vi "RSZVB Get Sweep Segment Name.vi"(8 "error in (no error)":errorcluster {"code" format="%.0x"}, 9 "Segment (1)":i32=1, 10 "Channel (1)":i32=1, 11 "VISA session":refnum<visa-resource-name>) -> (0 "error out":errorcluster {"code" format="%.0x"}, 2 "Name":string, 3 "dup VISA session":refnum<visa-resource-name>)   [LabVIEW 2011]
doc: "This VI returns the Name of the sweep segment no. <Seg>.\n\nRemote-control command(s):\n[SENSe<Ch>:]SEGMent<Seg>:NAME?"
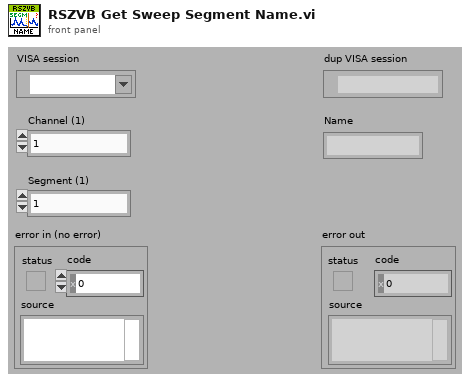
[diagram p1: front panel]
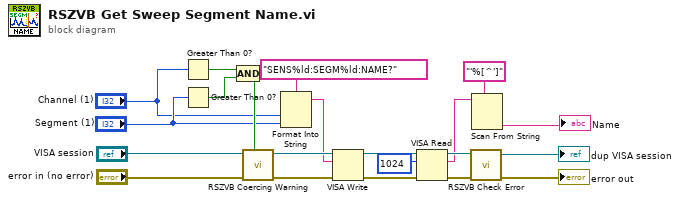
[diagram p0: block diagram]
diagram:
  n1 = Greater Than 0?(x="Channel (1)") -> (x > 0?=w16:bool)
  n2 = Greater Than 0?(x="Segment (1)") -> (x > 0?=w15:bool)
  n3 = Compound Arithmetic op=AND(w16, w15) -> (w18:bool)
  n4 = call "RSZVB Coercing Warning.vi"("In Range?"=w18, "error in (no error)"="error in (no error)", "VISA session"="VISA session") -> ("error out"=w19:errorcluster, "dup VISA session"=w20:refnum<visa-resource-name>)  [unwired: 7 in]
  n5 = Format Into String(format string="SENS%ld:SEGM%ld:NAME?", "Channel (1)", "Segment (1)") -> (resulting string=w17:string)  [unwired: 2 in, 1 out]
  n6 = VISA Write(VISA resource name=w20, write buffer=w17, error in (no error)=w19) -> (VISA resource name out=w11:refnum<visa-resource-name>, error out=w10:errorcluster)  [unwired: 1 out]
  n7 = VISA Read(VISA resource name=w11, byte count=u32 1024 ("byte count (0)"), error in (no error)=w10) -> (VISA resource name out=w13:refnum<visa-resource-name>, read buffer=w1:string, error out=w12:errorcluster)  [unwired: 1 out]
  n8 = call "RSZVB Check Error.vi"("error in (no error)"=w12, "VISA session"=w13) -> ("error out"=→"error out":errorcluster, "dup VISA session"=→"dup VISA session":refnum<visa-resource-name>)  [unwired: 8 in]
  n9 = Scan From String(format string="'%[^']", input string=w1) -> (output 1=→"Name":string)  [unwired: 3 in, 3 out]
